vi "Launch Hardware Interface.vi"(8 "error in (no error)":errorcluster, 11 "Tamagotchi Full Actor in":refnum<class "Tamagotchi Full Actor.lvclass">) -> (0 "error out":errorcluster, 3 "Tamagotchi Full Actor out":refnum<class "Tamagotchi Full Actor.lvclass">)   [LabVIEW 2026, in "Tamagotchi Full Actor.lvclass"]
uses:
  Tamagotchi Full Actor.lvclass
  C:/Program Files/National Instruments/LabVIEW 2026/vi.lib/ActorFramework/Actor/Actor.lvclass
  4_A2A Comms/Hardware Interface Actor/Hardware Interface Actor.lvclass
  <vilib>/ActorFramework/Actor/Actor.lvclass
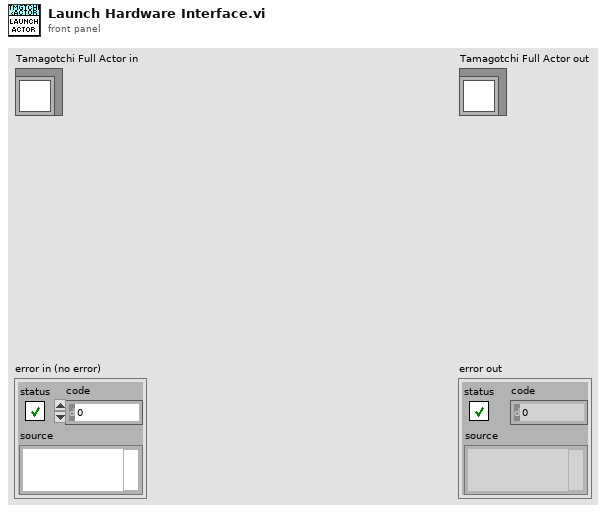
[diagram p1: front panel]
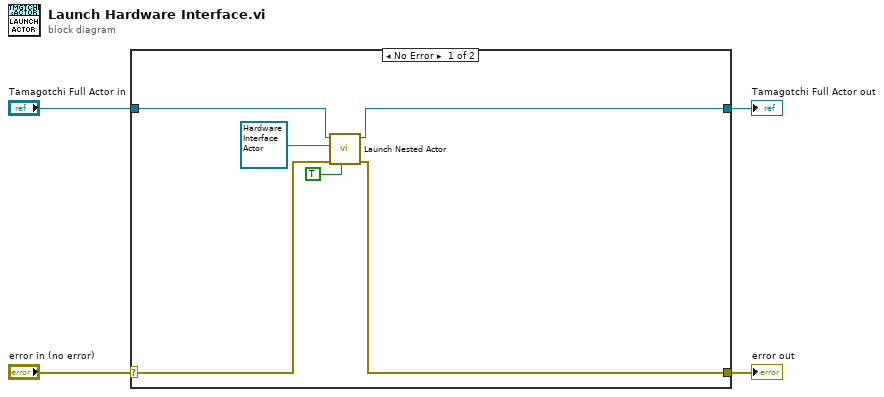
[diagram p0: block diagram]
diagram:
  n1 = case shown="No Error" "error in (no error)" {
    selector: "error in (no error)" -> [w6 w12]
    tunnel: [w5 w12] -> w3
    tunnel: [w10 w11] -> w1
    tunnel: "Tamagotchi Full Actor in" -> [w9 w11]
    frame No Error {
      n2 = call <vilib>:"Launch Nested Actor.vi"("Open Actor Core front panel? (F)"=TRUE, "error in (no error)"=w6, "Nested Actor"=refnum<class "Hardware Interface Actor.lvclass"> refnum ("Hardware Interface Actor.lvclass"), "Caller Actor in"=w9) -> ("error out"=w5:errorcluster, "Caller Actor out"=w10:refnum<class "Tamagotchi Full Actor.lvclass">)  [unwired: 5 in, 1 out]
    }
    frame Error {
    }
  }
  "error out" <- w3
  "Tamagotchi Full Actor out" <- w1
